vi "Memory Benchmark Async.vi"(8 "error in (no error)":errorcluster, 10 "copy sizes":u64[](array[numeric]), 11 "UI Pointers":T1) -> (0 "error out":errorcluster, 1 "peak index":i32, 2 "peak throughput":dbl, 3 "results":cluster{"X":dbl[], "Y":dbl[]})   [LabVIEW 2020]
uses:
  UI Pointers.ctl
  Source/Classes/Pointer/Stop/Stop Pointer.lvclass
  Source/Classes/Pointer/Pointer.lvclass
  Source/Classes/Pointer/Write I32.vi
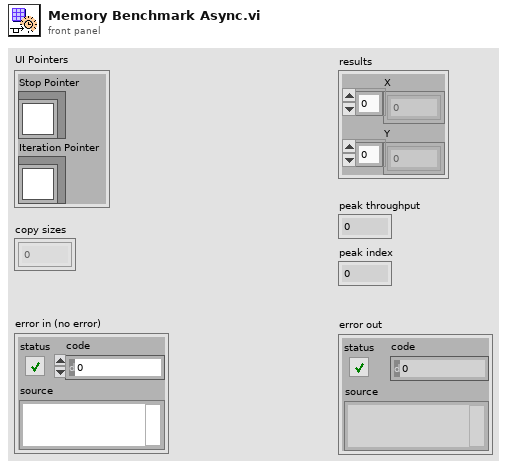
[diagram p1: front panel]
types:
  T1 = typedef "UI Pointers.ctl" = cluster{"Stop Pointer":refnum<class "Stop Pointer.lvclass">, "Iteration Pointer":refnum<class "Pointer.lvclass">}
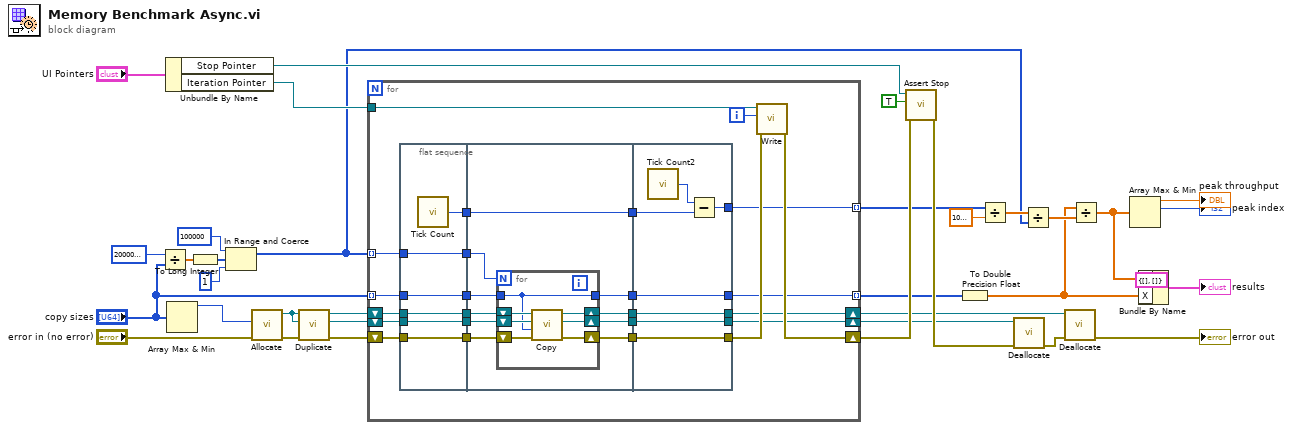
[diagram p0: block diagram]
diagram:
  n1 = Divide(x=u64 200000000, y="copy sizes") -> (x/y=w34:dbl[])
  n2 = Unbundle By Name("UI Pointers") -> ("Stop Pointer"=w8:refnum<class "Stop Pointer.lvclass">, "Iteration Pointer"=w7:refnum<class "Pointer.lvclass">)
  n3 = Array Max & Min(array="copy sizes") -> (max value=w28:u64)  [unwired: 3 out]
  n4 = To Long Integer(number=w34) -> (32bit integer=w33:i32[])
  n5 = In Range and Coerce(upper limit=100000, x=w33, lower limit=1) -> (coerced(x)=w2:i32[])  [unwired: 1 out]
  n6 = call "Allocate.vi"("error in (no error)"="error in (no error)", "size"=w28) -> ("error out"=w30:errorcluster, "Pointer out"=w29:refnum<class "Pointer.lvclass">)  [unwired: 8 in]
  n7 = call "Duplicate.vi"("error in (no error)"=w30, "new Pointer type"=w29, "Pointer in"=w29) -> ("error out"=w24:errorcluster, "new Pointer"=w27:refnum<class "Pointer.lvclass">, "Pointer out"=w26:refnum<class "Pointer.lvclass">)  [unwired: 6 in]
  n8 = for {
    shift-right: [w40] -> w19
    shift-left: w27 -> [w47]
    shift-right: [w38] -> w18
    shift-left: w26 -> [w46]
    shift-right: [w43] -> w20
    shift-left: w24 -> [w45]
    tunnel: [w36] -> w10 mode=indexing
    tunnel: "copy sizes" -> [w44] mode=indexing
    tunnel: [w37] -> w11 mode=indexing
    tunnel: w2 -> [w48] mode=indexing
    tunnel: w7 -> [w39]
    i -> [w41]
    n9 = flat-sequence {
      tunnel: [w65] -> w59
      tunnel: [w64] -> w58
      tunnel: [w63] -> w57
      tunnel: [w62] -> w56
      tunnel: [w61] -> w55
      tunnel: [w60] -> w54
      tunnel: w46 -> [w65]
      tunnel: w47 -> [w64]
      tunnel: w45 -> [w63]
      tunnel: w44 -> [w62]
      tunnel: w48 -> [w61]
      tunnel: w59 -> [w75]
      tunnel: w58 -> [w66]
      tunnel: w57 -> [w74]
      tunnel: w56 -> [w73]
      tunnel: w55 -> [w69]
      tunnel: w54 -> [w68]
      tunnel: [w68] -> w53
      tunnel: [w72] -> w52
      tunnel: [w71] -> w51
      tunnel: [w70] -> w50
      tunnel: [w67] -> w49
      tunnel: w53 -> [w88]
      tunnel: w52 -> [w87]
      tunnel: w51 -> [w86]
      tunnel: w50 -> [w85]
      tunnel: w49 -> [w84]
      tunnel: [w87] -> w42
      tunnel: [w86] -> w38
      tunnel: [w85] -> w40
      tunnel: [w84] -> w37
      tunnel: [w83] -> w36
      frame #0 {
        n10 = call "Tick Count"() -> ("Tick Count(uSec)"=w60:u32)
      }
      frame #1 {
        n11 = for {
          N: w69 -> [_]
          shift-right: [w79] -> w72
          shift-left: w74 -> [w80]
          shift-right: [w78] -> w71
          shift-left: w75 -> [w82]
          shift-right: [w77] -> w70
          shift-left: w66 -> [w81]
          tunnel: w73 -> [w76]
          tunnel: [w76] -> w67
          n12 = call "Copy.vi"("error in (no error)"=w80, "size"=w76, "dst Pointer in"=w81, "src Pointer in"=w82) -> ("error out"=w79:errorcluster, "dst Pointer out"=w77:refnum<class "Pointer.lvclass">, "src Pointer out"=w78:refnum<class "Pointer.lvclass">)  [unwired: 4 in, 1 out]
        }
      }
      frame #2 {
        n13 = call "Tick Count2"() -> ("Tick Count(uSec)"=w89:u32)
        n14 = Subtract(x=w89, y=w88) -> (x-y=w83:u32)
      }
    }
    n15 = call-poly "Write.vi"("error in (no error)"=w42, "value"=w41, "Pointer in"=w39) -> ("error out"=w43:errorcluster)  [unwired: 5 in, 3 out]
  }
  n16 = call "Assert Stop.vi"("error in (no error)"=w20, "stop (F)"=TRUE, "Stop Pointer in"=w8) -> ("error out"=w22:errorcluster)  [unwired: 6 in, 2 out]
  n17 = To Double Precision Float(number=w11) -> (double precision float=w4:dbl[])
  n18 = Divide(x=w10, y=1000000.0) -> (x/y=w3:dbl[])
  n19 = call "Deallocate.vi"("error in (no error)"=w22, "Pointer"=w19) -> ("error out"=w23:errorcluster)  [unwired: 8 in, 1 out]
  n20 = Divide(x=w3, y=w2) -> (x/y=w13:dbl[])
  n21 = call "Deallocate.vi"("error in (no error)"=w23, "Pointer"=w18) -> ("error out"=→"error out":errorcluster)  [unwired: 8 in, 1 out]
  n22 = Divide(x=w4, y=w13) -> (x/y=w16:dbl[])
  n23 = Array Max & Min(array=w16) -> (max value=→"peak throughput":dbl, max index (indices)=→"peak index":i32)  [unwired: 2 out]
  n24 = Bundle By Name(cluster=cluster{"X":dbl[], "Y":dbl[]} {"X"=[], "Y"=[]}, "Y"=w16, "X"=w4) -> (→"results":cluster{"X":dbl[], "Y":dbl[]})
